vi "set thread pool if null.vi"(10 "dispatcher":refnum<data-value>, 11 "task in":refnum<class "task.lvclass">) -> (3 "task out":refnum<class "task.lvclass">)   [LabVIEW 2013, in "task.lvclass"]
uses:
  task.lvclass
  dispatcher/thread pool.lvclass
  task.lvclass/task.ctl
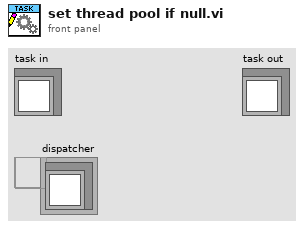
[diagram p1: front panel]
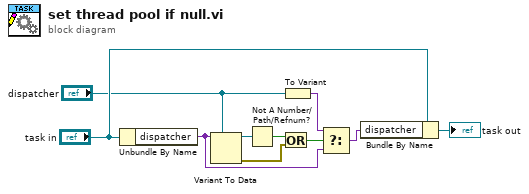
[diagram p0: block diagram]
diagram:
  n1 = Unbundle By Name("task in") -> ("dispatcher"=w4:variant)
  n2 = Variant To Data(type="dispatcher", Variant=w4) -> (data=w8:refnum<data-value>, error out=w6:errorcluster)  [unwired: 1 in]
  n3 = Not A Number/Path/Refnum?(number/path/refnum=w8) -> (NaN/Path/Refnum?=w7:bool)
  n4 = Or(x=w7, y=w6) -> (x .or. y?=w5:bool)
  n5 = To Variant(anything="dispatcher") -> (Variant=w2:variant)
  n6 = Select(t=w2, s=w5, f=w4) -> (s? t:f=w1:variant)
  n7 = Bundle By Name(cluster="task in", "dispatcher"=w1) -> (→"task out":refnum<class "task.lvclass">)
